vi "MB Ethernet Is Address Valid.vi"(8 "error in (no error)":errorcluster, 10 "Valid IP Addresses":string[](array[string]), 11 "IP Address":string) -> (0 "error out":errorcluster, 3 "IP Valid":bool)   [LabVIEW 2023, in "Voegtlin_NI_SMART_Modbus_Drivers.lvlib"]
uses:
  Voegtlin_NI_SMART_Modbus_Drivers.lvlib
panel:
  # "VI Name: IVB Ethernet Is Address Valid.vi\nPurpose: Verifies if the IP Address can be masked by one of the\naddresses provided in the Valid IP Addresses array."
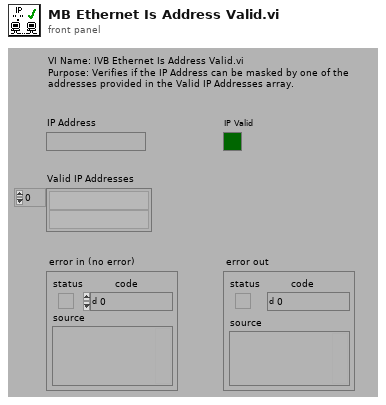
[diagram p1: front panel]
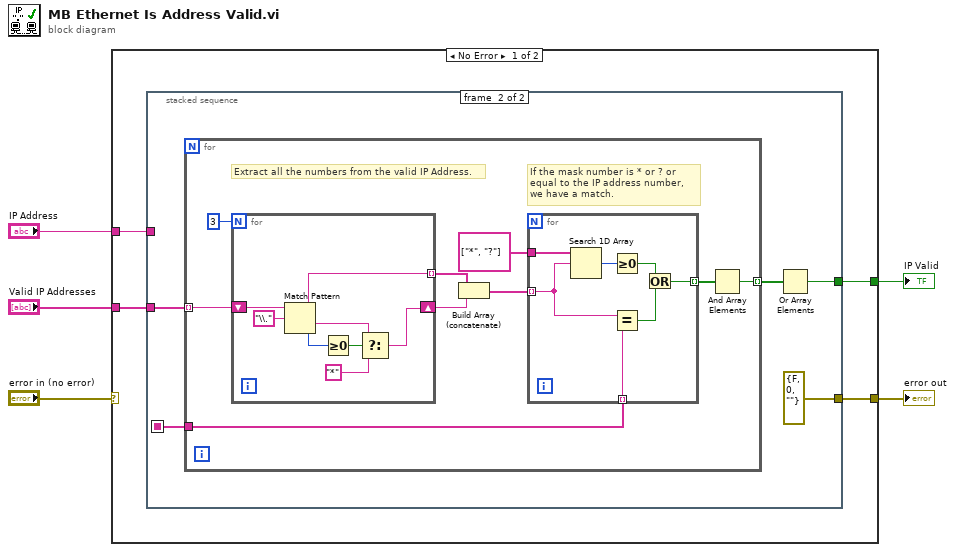
[diagram p0: block diagram]
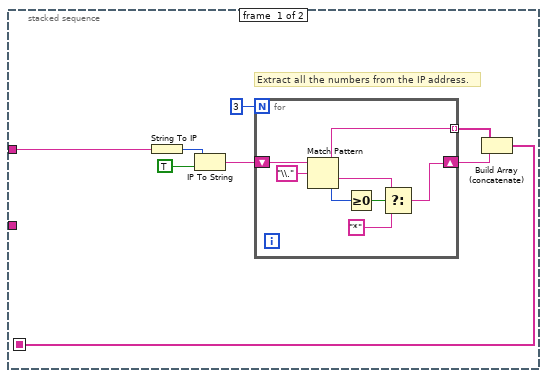
[diagram p2: hidden frame]
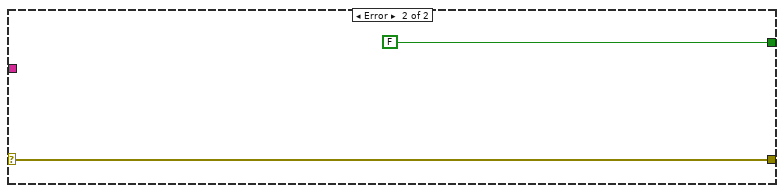
[diagram p3: hidden frame]
diagram:
  n1 = case shown="No Error" "error in (no error)" {
    selector: "error in (no error)" -> [_ w55]
    tunnel: "Valid IP Addresses" -> [w9 _]
    tunnel: "IP Address" -> [w6 _]
    tunnel: [w8 FALSE] -> w3
    tunnel: [w7 w55] -> w1
    frame No Error {
      n2 = stacked-sequence {
        seq-local: [w14 _] -> [_ w26]
        tunnel: w9 -> [_ w30]
        tunnel: [_ w29] -> w8
        tunnel: [_ errorcluster {"status"=FALSE, "code"=0, "source"=""} ("error IO")] -> w7
        tunnel: w6 -> [w11 _]
        frame #0 {
          # "Extract all the numbers from the IP address."
          n3 = String To IP(1:w11) -> (0:w13:u32)
          n4 = IP To String(1:TRUE ("dot notation? (F)"), 2:w13) -> (0:w10:string)
          n5 = for {
            N: 3 -> [_]
            shift-right: [w19] -> w16
            shift-left: w10 -> [w25]
            tunnel: [w18] -> w15 mode=indexing
            n6 = Match Pattern(string=w25, regular expression="\\.") -> (before substring=w18:string, after substring=w21:string, offset past match=w23:i32)  [unwired: 2 out]
            n7 = Greater Or Equal To 0?(x=w23) -> (x >= 0?=w22:bool)
            n8 = Select(t=w21, s=w22, f="*") -> (s? t:f=w19:string)
          }
          n9 = Build Array (concatenate)(w15, w16) -> (w14:string[])
        }
        frame #1 {
          n10 = for {
            tunnel: w30 -> [w31] mode=indexing
            tunnel: [w33] -> w28 mode=indexing
            tunnel: w26 -> [w32]
            # "If the mask number is * or ? or equal to the IP address number, we have a match."
            # "Extract all the numbers from the valid IP Address."
            n11 = for {
              N: 3 -> [_]
              shift-right: [w48] -> w38
              shift-left: w31 -> [w54]
              tunnel: [w47] -> w37 mode=indexing
              n12 = Match Pattern(string=w54, regular expression="\\.") -> (before substring=w47:string, after substring=w50:string, offset past match=w52:i32)  [unwired: 2 out]
              n13 = Greater Or Equal To 0?(x=w52) -> (x >= 0?=w51:bool)
              n14 = Select(t=w50, s=w51, f="*") -> (s? t:f=w48:string)
            }
            n15 = Build Array (concatenate)(w37, w38) -> (w34:string[])
            n16 = for {
              tunnel: [w42] -> w35 mode=indexing
              tunnel: string[] ["*", "?"] -> [w45]
              tunnel: w34 -> [w41] mode=indexing
              tunnel: w32 -> [w40] mode=indexing
              n17 = Search 1D Array(1D array=w45, element=w41) -> (index of element=w46:i32)  [unwired: 1 out]
              n18 = Greater Or Equal To 0?(x=w46) -> (x >= 0?=w44:bool)
              n19 = Equal?(x=w41, y=w40) -> (x = y?=w43:bool)
              n20 = Or(x=w44, y=w43) -> (x .or. y?=w42:bool)
            }
            n21 = And Array Elements(Boolean array=w35) -> (logical AND=w33:bool)
          }
          n22 = Or Array Elements(Boolean array=w28) -> (logical OR=w29:bool)
        }
      }
    }
    frame Error {
    }
  }
  "IP Valid" <- w3
  "error out" <- w1
